vi "Device Select.vi"(8 "error in":errorcluster, 10 "SQL query":string="SELECT distinct DeviceName \nFROM\nltt.daq_configuration\n Where ChannelType='PWM_Output' and Enabled=1;", 11 "NI PWM Output in":refnum<class "NI PWM Output.lvclass">) -> (0 "error out":errorcluster, 3 "NI PWM Output out":refnum<class "NI PWM Output.lvclass">)   [LabVIEW 2023, in "HardwareAbstractionLayer_LVOOP.lvlib" / "NI PWM Output.lvclass"]
doc: "This VI Selected Device"
uses:
  NI PWM Output.lvclass
  NI PWM Output.lvclass/NI PWM Output.ctl
  Database/Database.lvclass
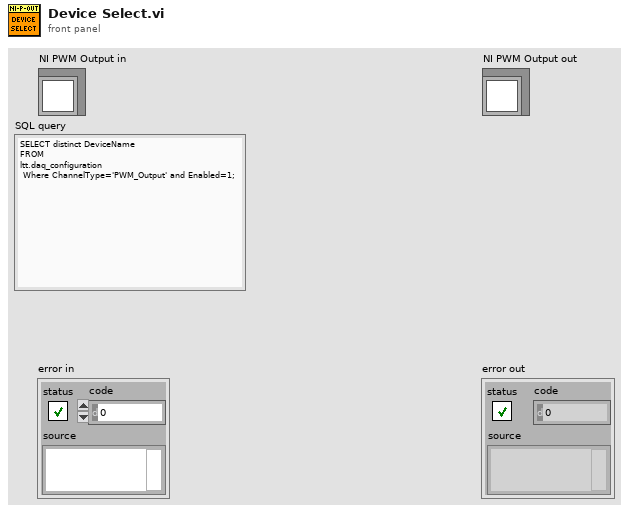
[diagram p1: front panel]
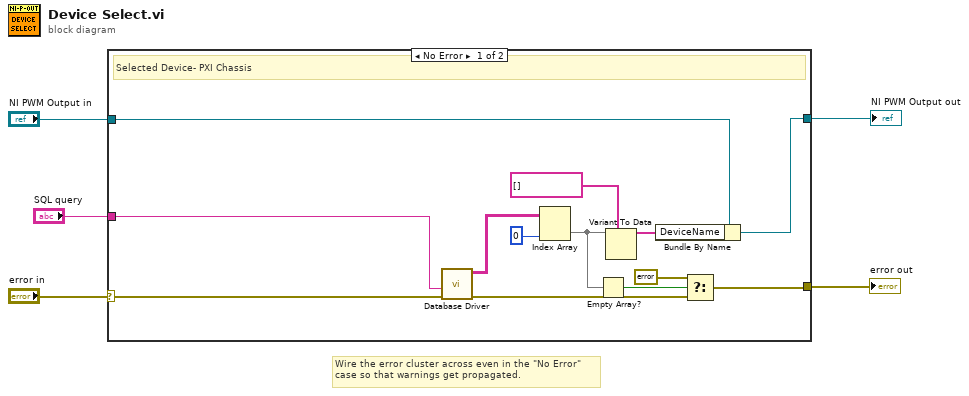
[diagram p0: block diagram]
diagram:
  # "Wire the error cluster across even in the \"No Error\"\ncase so that warnings get propagated."
  n1 = case shown="No Error" "error in" {
    selector: "error in" -> [w12 w20]
    tunnel: [w8 w20] -> w4
    tunnel: [w17 w19] -> w2
    tunnel: "NI PWM Output in" -> [w18 w19]
    tunnel: "SQL query" -> [w6 _]
    frame No Error {
      # "Selected Device- PXI Chassis"
      n2 = call "Database Driver.vi"("error in"=w12, "SQL query"=w6) -> ("error out"=w9:errorcluster, "data"=w13:string[][])  [unwired: 6 in, 2 out]
      n3 = Index Array(array=w13, index (col)=0 ("disabled index (col)")) -> (element=w11:string[])  [unwired: 1 in]
      n4 = Empty Array?(array=w11) -> (empty?=w10:bool)
      n5 = Variant To Data(type=tag[] [] ("DeviceName"), Variant=w11) -> (data=w14:tag[])  [unwired: 1 in, 1 out]
      n6 = Bundle By Name(cluster=w18, "DeviceName"=w14) -> (w17:refnum<class "NI PWM Output.lvclass">)
      n7 = Select(t=errorcluster {"status"=TRUE, "code"=0, "source"="Database does not contains device which is query."}, s=w10, f=w9) -> (s? t:f=w8:errorcluster)
    }
    frame Error {
    }
  }
  "error out" <- w4
  "NI PWM Output out" <- w2
